vi "q3 npr ncr.vi"() -> ()   [LabVIEW 2025]
panel:
  out "nCr":dbl
  out "nPr":dbl
  in  "r":dbl
  in  "n":dbl
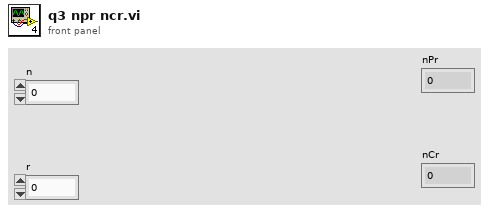
[diagram p1: front panel]
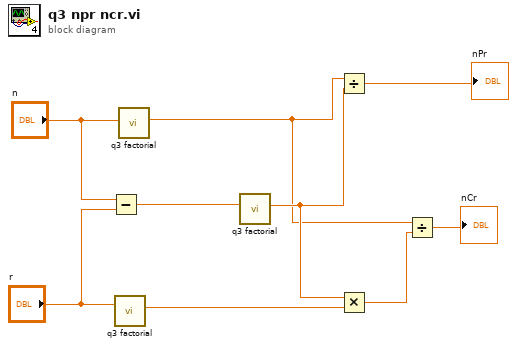
[diagram p0: block diagram]
diagram:
  n1 = Subtract(x="n", y="r") -> (x-y=w7:dbl)
  n2 = call "q3 factorial.vi"("n"="r") -> ("n!"=w5:dbl)  [unwired: 10 in]
  n3 = call "q3 factorial.vi"("n"="n") -> ("n!"=w3:dbl)  [unwired: 10 in]
  n4 = call "q3 factorial.vi"("n"=w7) -> ("n!"=w4:dbl)  [unwired: 10 in]
  n5 = Divide(x=w3, y=w4) -> (x/y=→"nPr":dbl)
  n6 = Multiply(x=w4, y=w5) -> (x*y=w2:dbl)
  n7 = Divide(x=w3, y=w2) -> (x/y=→"nCr":dbl)
